vi "MatLab_Full.vi"(2 "Levels":dbl=5.0, 3 "input Array":dbl[][](array[numeric]), 4 "WaveletType":string="db04") -> (0 "dominantFrequencies Array":string[](array[string]), 1 "dominantFrequencies":dbl[](array[numeric]))   [LabVIEW 2023]
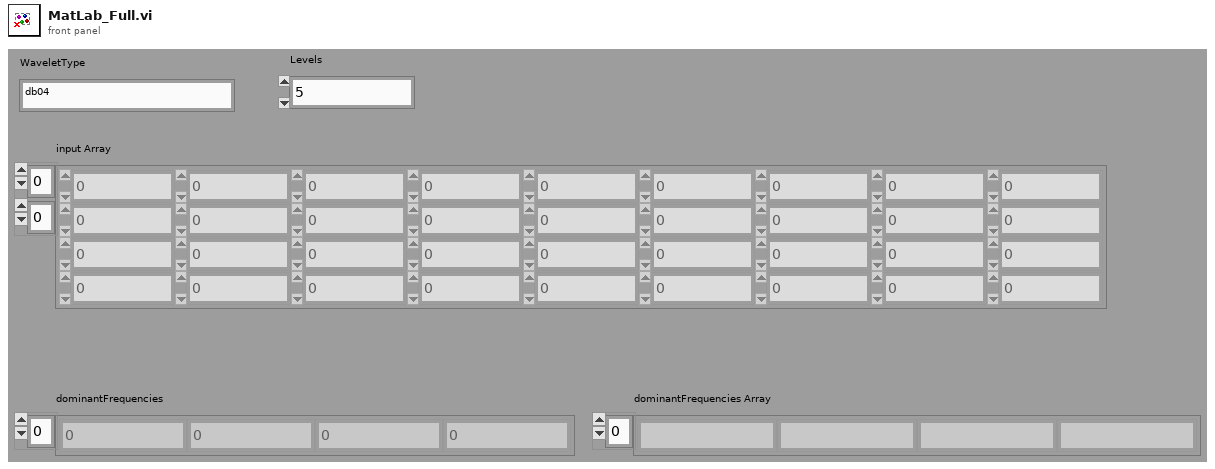
[diagram p1: front panel]
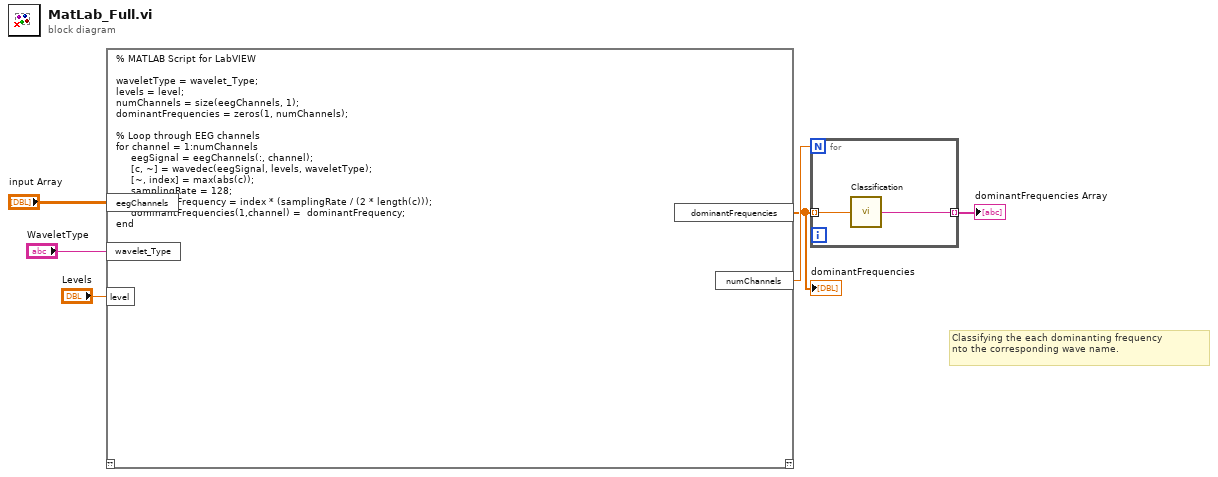
[diagram p0: block diagram]
diagram:
  # "Classifying the each dominanting frequency \nnto the corresponding wave name."
  n1 = script code="% MATLAB Script for LabVIEW\n\nwaveletType = wavelet_Type;\nlevels = level;\nnumChannels = size(eegChannels, 1);\ndominantFrequencies = zeros(1, numChannels);\n\n% Loop through EEG channels\nfor channel = 1:numChannels\n     eegSignal = eegChannels(:, channel);\n     [c, ~] = wavedec(eegSignal, levels, waveletType);\n     [~, index] = max(abs(c));\n     samplingRate = 128;\n     dominantFrequency = index * (samplingRate / (2 * length(c)));\n     dominantFrequencies(1,channel) =  dominantFrequency;\nend"("eegChannels"="input Array", "wavelet_Type"="WaveletType", "level"="Levels") -> ("dominantFrequencies"=w1:dbl[], "numChannels"=w3:dbl)  [unwired: 1 in, 1 out]
  "dominantFrequencies" <- w1
  n2 = for {
    N: w3 -> [_]
    tunnel: w1 -> [w8] mode=indexing
    tunnel: [w7] -> w2 mode=indexing
    n3 = call "Classification.vi"("Numeric"=w8) -> ("Detected Wave"=w7:string)
  }
  "dominantFrequencies Array" <- w2
